vi "PXIe_1082_Find_Hardware.vi"(8 "error in (no error)":errorcluster, 10 "Search Device":string) -> (0 "error out":errorcluster, 2 "Is Present ?":bool, 3 "PXI Devices":string[][](table))   [LabVIEW 2024]
doc: "This VI inits a waveform generation session for the AO6711 board.\n1. The physical channels are selected as Analog Outputs.\n2. Init values are immediately written to the outputs.\n3. The board is inialized to wait for pulse triggers coming from an external source, i.e. the Trigger Source, and to deliver a finite number of samples.\n4. The samples have to be stored in on-board memory in a next VI."
uses:
  <vilib>/nisyscfg/Close (System).vi
  <resource>/objmgr/nicontrollersysapi.rc
  <vilib>/nisyscfg/nisyscfg.lvlib
  <resource>/objmgr/pxisysapi.rc
panel:
  out "Available":bool[](array[boolean])
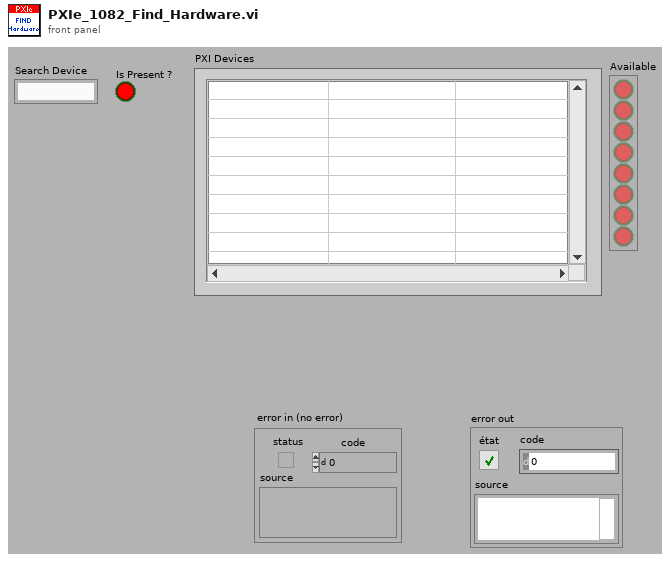
[diagram p1: front panel]
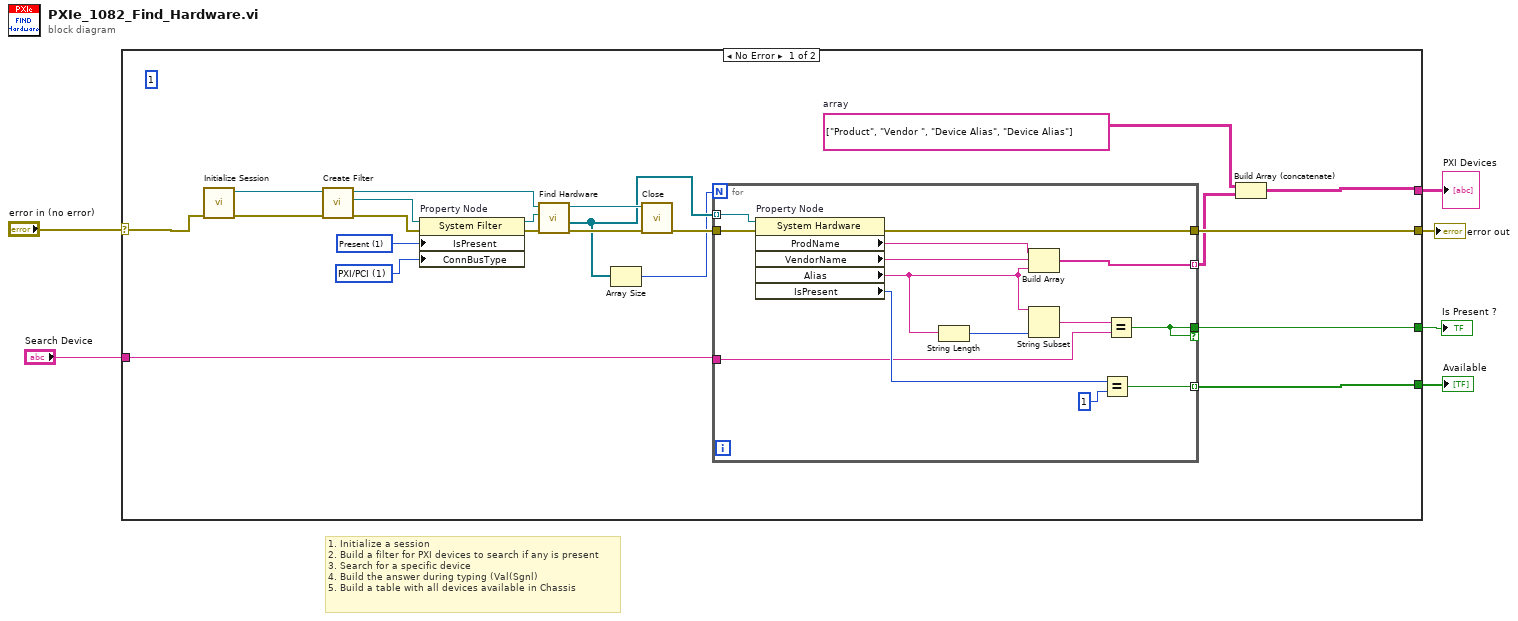
[diagram p0: block diagram]
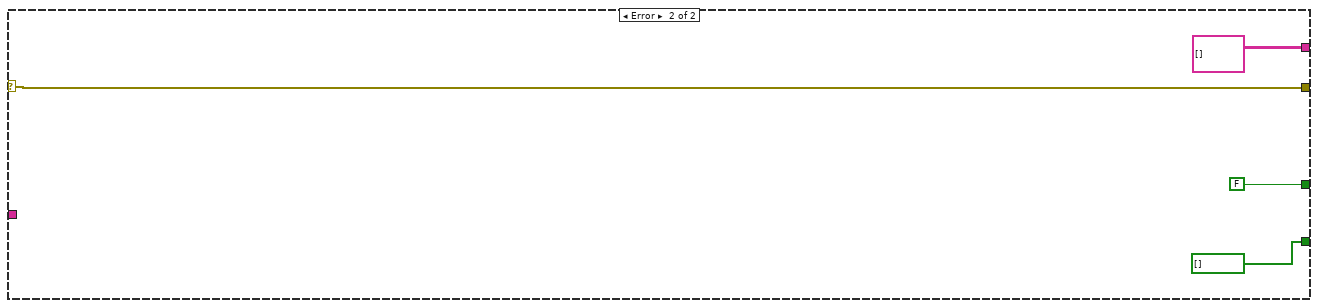
[diagram p2: hidden frame]
diagram:
  # "1. Initialize a session\n2. Build a filter for PXI devices to search if any is present\n3. Search for a specific device\n4. Build the answer during typing (Val(Sgnl)\n5. Build a table with all devices available in Chassis"
  n1 = case shown="No Error" "error in (no error)" {
    selector: "error in (no error)" -> [w24 w46]
    tunnel: [w28 w46] -> w6
    tunnel: [w25 string[][] []] -> w4
    tunnel: [w27 bool[] []] -> w3
    tunnel: [w26 FALSE] -> w2
    tunnel: "Search Device" -> [w23 _]
    frame No Error {
      w9 = u32 1 items=["BuiltIn/System", "PXI/PCI", "USB", "GPIB", "VXI", "Serial", "TCP/IP", "cRIO", "SCXI", "cDAQ", "SwitchBlock", "SCC", "FireWire", "Accessory", "CAN", "SwitchBlock Device", "SLSC"] ("Devices & Chassis:Connects To Bus Type")
      w10 = 1 items=["Initializing"=-2, "Unknown"=-1, "Not Present"=0, "Present"=1] ("Devices & Chassis:Is Present")
      w22 = string[][] [["Product", "Vendor ", "Device Alias", "Device Alias"]]  # array
      (unwired) 1
      n2 = call <vilib>:"Initialize Session.vi"("error in (no error)"=w24) -> ("error out"=w14:errorcluster, "Session out"=w13:refnum<k21>)  [unwired: 9 in]
      n3 = call <vilib>:"Create Filter.vi"("error in (no error)"=w14, "Session in"=w13) -> ("error out"=w11:errorcluster, "Filter out"=w12:refnum<k20>, "Session out"=w17:refnum<k21>)  [unwired: 7 in]
      n4 = property on="Property Node" class="System Filter"(reference=w12, error in=w11, "IsPresent"=w10, "ConnBusType"=w9) -> (reference out=w16:refnum<k20>, error out=w15:errorcluster)
      n5 = call <vilib>:"Find Hardware.vi"("error in (no error)"=w15, "Filter in"=w16, "Session in"=w17) -> ("error out"=w18:errorcluster, "Resources out"=w8:refnum<k20>[], "Session out"=w19:refnum<k21>)  [unwired: 5 in, 1 out]
      n6 = Array Size(array=w8) -> (size(s)=w7:i32)
      n7 = call-poly <vilib>:"Close.vi"("error in (no error)"=w18, "Session in"=w19) -> ("error out"=w20:errorcluster)  [unwired: 9 in]
      n8 = for {
        N: w7 -> [_]
        tunnel: w8 -> [w41] mode=indexing
        tunnel: w20 -> [w42]
        tunnel: [w39] -> w21 mode=indexing
        tunnel: [w36] -> w28
        tunnel: [w33] -> w27 mode=indexing
        tunnel: [w31] -> w26 if=w31
        tunnel: w23 -> [w30]
        n9 = property on="Property Node" class="System Hardware"(reference=w41, error in=w42) -> (error out=w36:errorcluster, "ProdName"=w35:string, "VendorName"=w40:string, "Alias"=w29:string, "IsPresent"=w32:i32)  [unwired: 1 out]
        n10 = String Length(string=w29) -> (length=w38:i32)
        n11 = Build Array "Build Array"(w35, w40, w29) -> (w39:string[])
        n12 = String Subset(string=w29, length (rest)=w38) -> (substring=w37:string)  [unwired: 1 in]
        n13 = Equal?(x=w32, y=1) -> (x = y?=w33:bool)
        n14 = Equal?(x=w37, y=w30) -> (x = y?=w31:bool)
      }
      n15 = Build Array (concatenate) "Build Array"(w22, w21) -> (w25:string[][])
    }
    frame Error {
    }
  }
  "error out" <- w6
  "PXI Devices" <- w4
  "Available" <- w3
  "Is Present ?" <- w2
